vi "m1m3_issueCommand_ApplyAberrationByForces.vi"(8 "error in (no error)":errorcluster, 11 "command_ApplyAberrationByForces_Ctl":T1) -> (0 "error out":errorcluster, 2 "function return":i32, 3 "command_ApplyAberrationByForces_Ctl out":T1)   [LabVIEW 2016, in "SALLV_m1m3.lvlib"]
doc: "int m1m3_shm_issueCommand_ApplyAberrationByForcesLV(m1m3_command_ApplyAberrationByForcesLV *command_ApplyAberrationByForces_Ctl );"
uses:
  SALLV_m1m3.lvlib
  DataTypes/command_ApplyAberrationByForces.ctl
  SALLV_m1m3.so
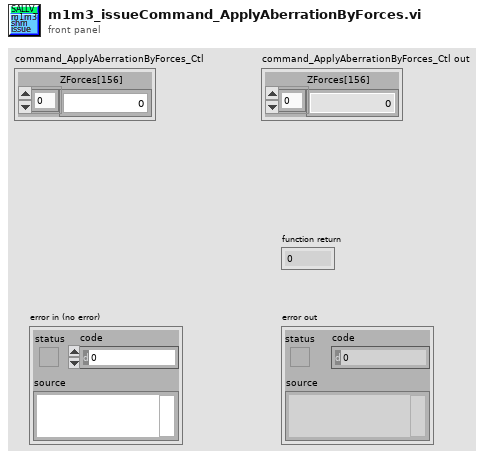
[diagram p1: front panel]
types:
  T1 = typedef "SALLV_m1m3.lvlib/command_ApplyAberrationByForces.ctl" = cluster{"ZForces[156]":dbl[]}
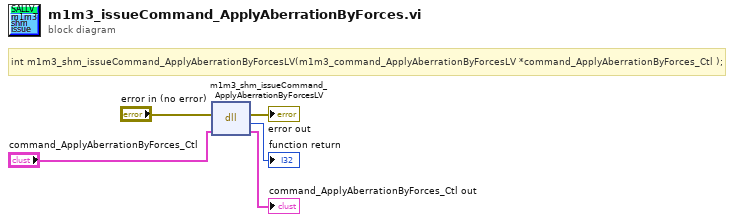
[diagram p0: block diagram]
diagram:
  # "int m1m3_shm_issueCommand_ApplyAberrationByForcesLV(m1m3_command_ApplyAberrationByForcesLV *command_ApplyAberrationByForces_Ctl );"
  n1 = dll-call lib="opt/CODE/SALLV_m1m3/SALLV_m1m3.*" fn="m1m3_shm_issueCommand_ApplyAberrationByForcesLV"(error in="error in (no error)", "command_ApplyAberrationByForces_Ctl"="command_ApplyAberrationByForces_Ctl") -> (error out=→"error out":errorcluster, →"function return":i32, "command_ApplyAberrationByForces_Ctl"=→"command_ApplyAberrationByForces_Ctl out":T1)  [unwired: 2 in, 1 out]
